vi "Periodic Tasks.vi"(8 "error in":errorcluster) -> ()   [LabVIEW 2015]
doc: "This VI runs in parallel to other tasks. It can contain as many user-defined periodic loops as you need. These can carry out PID or other sorts of timed response."
uses:
  PID Constants.ctl
  DriveTypes.ctl
  <vilib>/Rock Robotics/WPI/DriverStation/WPI_DriverStationAllianceInfo.ctl
  <vilib>/Rock Robotics/WPI/DriverStation/WPI_DriverStationPositionInfo.ctl
  IMUType.ctl
  <userlib>/836-Library/Drive/Drive Code/Drive Code Support/Drive Code PID Bundle.ctl
  <userlib>/836-Library/Pneumatics/Support Code/Solenoid Configure.ctl
  <userlib>/836-Library/Pneumatics/Support Code/Pneumatics Configuration.ctl
  <userlib>/836-Library/Pneumatics/Support Code/Feedback Method.ctl
  <vilib>/Platform/TimedLoop/XDataNode/timing_clust.ctl
  <vilib>/Platform/TimedLoop/XDataNode/nitl_modes.ctl
  <vilib>/Platform/TimedLoop/XDataNode/wakeup.ctl
  <userlib>/836-Library/System/TDMSv2/TDMS Channel Info.ctl
  <userlib>/836-Library/System/TDMSv2/TDMS RT FIFO Packet.ctl
  <vilib>/Rock Robotics/WPI/Utilities/WPI_GetSetVariantRefNum.vi
  <vilib>/Rock Robotics/Network Tables/NT Write Number.vi
  <vilib>/Rock Robotics/Network Tables/NT Write Boolean.vi
  <vilib>/platform/TimedLoop/XDataNode/XDataNode.xnode
  <vilib>/addons/control/pid/NI_PID_pid.lvlib
  <vilib>/Platform/TimedLoop/XDataNode/XDNodeRunTimeDep.lvlib
  <vilib>/addons/control/pid/pid.llb/PID Output Rate Limiter (DBL).vi
panel:
  out "IMU Type":T1
  out "Analog Pitch Gyro 2":dbl(graph)=-229.6875
  in  "Alt imu":bool
  in  "PImu fail":bool
  in  "Reload QCP":bool
  out "Position":T2
  out "Alliance":T3
  in  "Tab Control":enum32{"Drive Test", "IMU", "Drive", "IMU ALT"}(tab)=enum."Drive"
  out "Distance":T4(graph)
  out "Angle":cluster{"Angle Setpoint":dbl, "Yaw":dbl}(graph)={"Angle Setpoint"=87.11416811253483, "Yaw"=3.4375}
  in  "Negates":T5={"negate turn"=TRUE, "negate throttle"=FALSE}
  in  "Throttle Scale":dbl(knob)=0.6332538458134985 scale=0.0..1.0
  in  "Distance Delta":dbl=10.0
  in  "Angle Delta":dbl(knob)=83.67666811253483 scale=-100.0..100.0
  in  "output rate (EGU/min)":dbl(knob)=125.7747299198201 scale=0.0..200.0
  in  "Angle Wrap":bool
  in  "Eval Period (sec)":dbl(knob)=0.503724380465646 scale=0.0..1.0
  in  "tol":dbl=0.5 format="%#_13g"
  out "Shoot":bool
  in  "Period":i64=20
  out "Late?":bool
  out "Delta Angle Remaining":dbl=83.67666811253483
  in  "output range":cluster{"output high":dbl, "output low":dbl}={"output high"=1.0, "output low"=-1.0}
  out "Delta Angle Remaining 3":dbl
  out "Drive Mode 2":T6
  in  "PID Constants":T7={"Drive Distance PID"={"proportional gain (Kc)"=0.2, "integral time (Ti, min)"=0.0, "derivative time (Td, min)"=0.001}, "Drive Straight PID"={"proportional gain (Kc)"=0.035, "integral time (Ti, min)"=0.0, "derivative time (Td, min)"=0.0008}, "TurnPID"={"proportional gain (Kc)"=0.07, "integral time (Ti, min)"=0.005, "derivative time (Td, min)"=0.0008}, "Hold Position PID"={"proportional gain (Kc)"=0.2, "integral time (Ti, min)"=0.02, "derivative time (Td, min)"=0.001}} {"Hold Position PID"."derivative time (Td, min)" format="%.10f"; "Hold Position PID"."integral time (Ti, min)" format="%.8f"; "Hold Position PID"."proportional gain (Kc)" format="%.3f"; "TurnPID"."derivative time (Td, min)" format="%.6f"; "TurnPID"."integral time (Ti, min)" format="%.10f"; "TurnPID"."proportional gain (Kc)" format="%.6f"; "Drive Straight PID"."derivative time (Td, min)" format="%.6f"; "Drive Straight PID"."integral time (Ti, min)" format="%.10f"; "Drive Straight PID"."proportional gain (Kc)" format="%.6f"; "Drive Distance PID"."derivative time (Td, min)" format="%.10f"; "Drive Distance PID"."integral time (Ti, min)" format="%.8f"; "Drive Distance PID"."proportional gain (Kc)" format="%.3f"}
  out "M":T8={"Boolean"=FALSE, "Boolean 2"=FALSE, "Boolean 3"=FALSE, "Boolean 4"=TRUE}
  out "A":T8={"Boolean"=FALSE, "Boolean 2"=FALSE, "Boolean 3"=TRUE, "Boolean 4"=FALSE}
  out "G":T8={"Boolean"=TRUE, "Boolean 2"=FALSE, "Boolean 3"=FALSE, "Boolean 4"=FALSE}
  out "S":T8={"Boolean"=FALSE, "Boolean 2"=FALSE, "Boolean 3"=FALSE, "Boolean 4"=TRUE}
  out "Analog Yaw Gyro":dbl(graph)=-229.6875
  in  "Read Enable":T9={"Cal Status"=TRUE, "Orientation"=TRUE, "Gyro"=FALSE, "Accelerometer"=FALSE, "Quanterion"=FALSE, "Accel Mode"=enum."Linear", "Magnetometer"=FALSE}
  out "Yaw":dbl(graph)=37.4375
  out "Pitch":dbl(graph)=1.75
  out "Roll":dbl(graph)=0.5
  out "X Acc":dbl
  out "Y Acc":dbl
  out "Z Acc":dbl
  out "Anomaly":bool
  in  "Earth Field (uT)":cluster{"Earth":dbl, "Tolerance":dbl}={"Earth"=51.0, "Tolerance"=5.0}
  out "Mag Vector":dbl
  out "IMUStatus":bool
  out "Late? 2":bool
  in  "Sensor Period":i64=20
  out "pitch":dbl=1.75
  in  "Offset 2":dbl(knob)=0.6008653928286186 scale=0.0..1.0
  in  "Dead Zone 2":dbl(knob)=0.09984207295572244 scale=0.0..1.0
  in  "Offset":dbl(knob)=0.267936230826254 scale=0.0..1.0
  in  "Dead Zone":dbl(knob)=0.10126960022109426 scale=0.0..1.0
  out "Left Encoder Distance":dbl=4402.950615
  out "Right Encoder Distance":dbl
  in  "Reset Encoders":bool
  out "pitch 2":dbl=1.75
  out "Mag Vector 2":dbl
  out "Anomaly 2":bool
  in  "Earth Field (uT) 2":cluster{"Earth":dbl, "Tolerance":dbl}={"Earth"=51.0, "Tolerance"=5.0}
  out "Z Acc 2":dbl
  out "Y Acc 2":dbl
  out "X Acc 2":dbl
  out "M 2":T8={"Boolean"=FALSE, "Boolean 2"=FALSE, "Boolean 3"=FALSE, "Boolean 4"=TRUE}
  out "A 2":T8={"Boolean"=FALSE, "Boolean 2"=FALSE, "Boolean 3"=TRUE, "Boolean 4"=FALSE}
  out "G 2":T8={"Boolean"=TRUE, "Boolean 2"=FALSE, "Boolean 3"=FALSE, "Boolean 4"=FALSE}
  out "S 2":T8={"Boolean"=FALSE, "Boolean 2"=FALSE, "Boolean 3"=FALSE, "Boolean 4"=TRUE}
  in  "Read Enable 2":T9={"Cal Status"=TRUE, "Orientation"=TRUE, "Gyro"=FALSE, "Accelerometer"=FALSE, "Quanterion"=FALSE, "Accel Mode"=enum."Linear", "Magnetometer"=FALSE}
  # "Bazemore\nStraight Gains\nP=0.035\nI=0.00\nD=0.0008"
  # "Cass\nHold Position\nGains\nP=0.2\nI=0.02\nD=0.001"
  # "Bazemore\nTurn Gains\nP=0.07\nI=0.005\nD=0.0008"
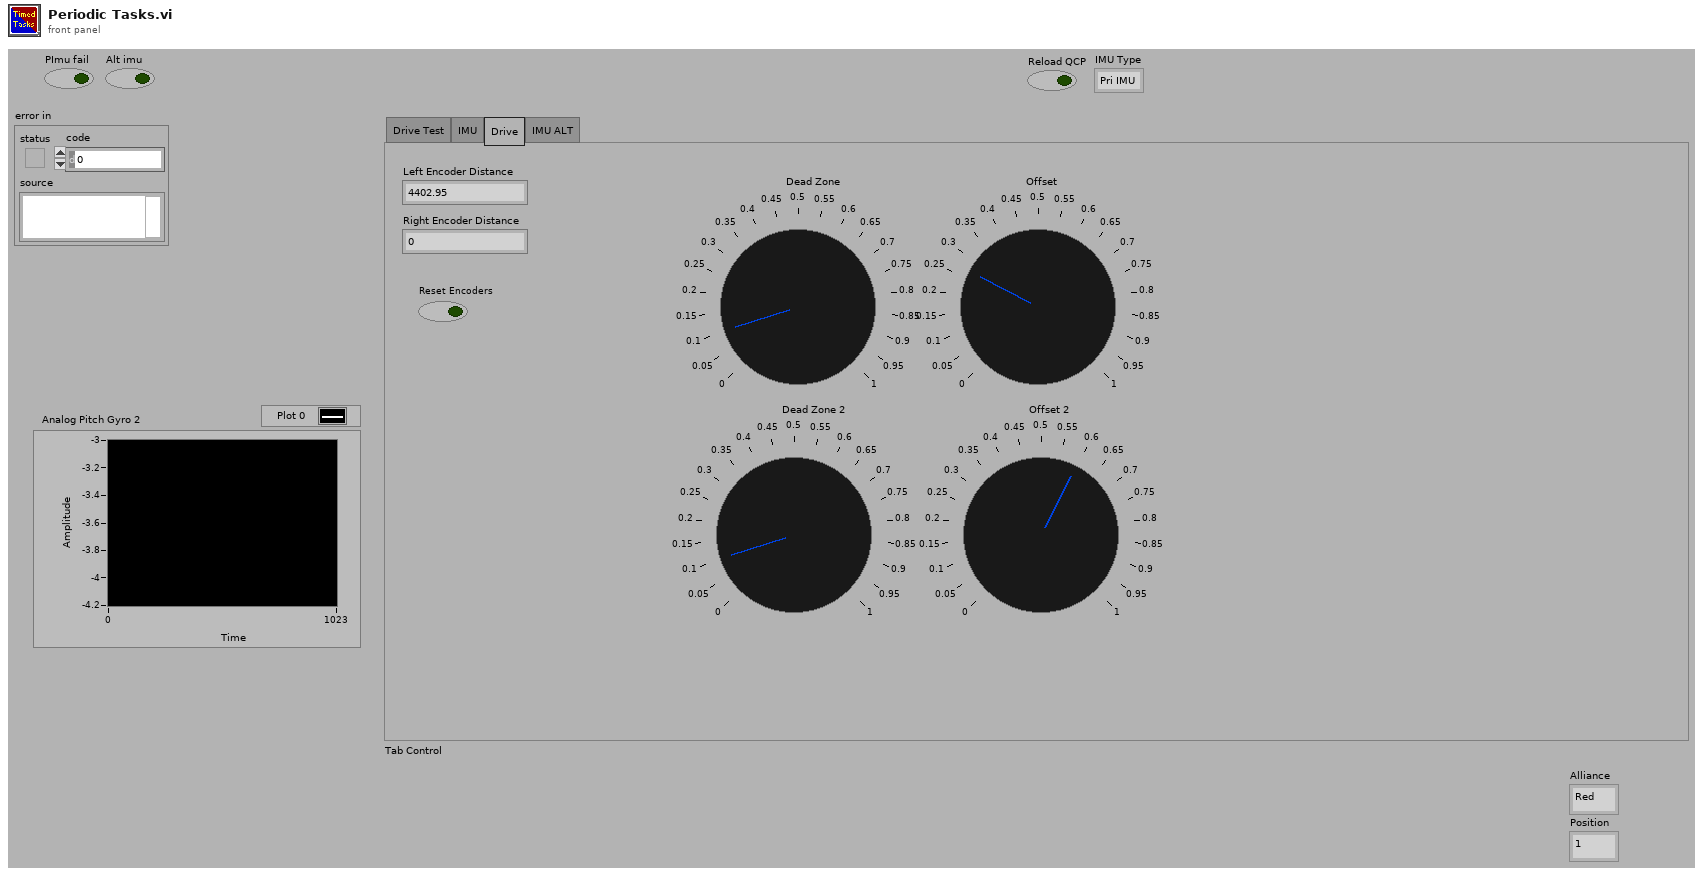
[diagram p1: front panel]
types:
  T1 = typedef "IMUType.ctl" = enum16{"Pri IMU", "Alt IMU", "Analog GYRO"}
  T2 = typedef "WPI_DriverStationPositionInfo.ctl" = enum16{"1", "2", "3"}
  T3 = typedef "WPI_DriverStationAllianceInfo.ctl" = enum16{"Red", "Blue", "Invalid"}
  T4 = cluster{"Distance Setpoint":dbl, "Desired Distance":dbl}
  T5 = cluster{"negate turn":bool, "negate throttle":bool}
  T6 = typedef "DriveTypes.ctl" = enum16{"Auto Turn", "Auto Straight", "Auto Vision Align"}
  T7 = typedef "PID Constants.ctl" = cluster{"Drive Distance PID":cluster{"proportional gain (Kc)":dbl, "integral time (Ti, min)":dbl, "derivative time (Td, min)":dbl}, "Drive Straight PID":cluster{"proportional gain (Kc)":dbl, "integral time (Ti, min)":dbl, "derivative time (Td, min)":dbl}, "TurnPID":cluster{"proportional gain (Kc)":dbl, "integral time (Ti, min)":dbl, "derivative time (Td, min)":dbl}, "Hold Position PID":cluster{"proportional gain (Kc)":dbl, "integral time (Ti, min)":dbl, "derivative time (Td, min)":dbl}}
  T8 = cluster{"Boolean":bool, "Boolean 2":bool, "Boolean 3":bool, "Boolean 4":bool}
  T9 = cluster{"Cal Status":bool, "Orientation":bool, "Gyro":bool, "Accelerometer":bool, "Quanterion":bool, "Accel Mode":enum8{"Raw Data", "Linear", "Gravity"}, "Magnetometer":bool}
  T10 = cluster{"Group":string, "Channel Names":string[]}[]
  T11 = typedef "TDMS Channel Info.ctl" = cluster{"TDMS Data":T12, "TDMS RT FIFO":refnum<k33>}
  T12 = typedef "TDMS RT FIFO Packet.ctl" = cluster{"Group/CMD":i32, "Channel":i32, "Data":dbl}
  T13 = cluster{"IMU Yaw":T11, "IMU Pitch":T11, "IMU Roll":T11, "Accel X":T11, "Accel Y":T11, "Accel Z":T11, "IMU Cal M":T11, "IMU Cal A":T11, "IMU Cal G":T11, "IMU Cal S":T11, "IMU Type":T11}
  T14 = typedef "Solenoid Configure.ctl" = cluster{"Normal Timing":T15, "Feedback Forward":T16, "Feedback Reverse":T16, "Analog Thresholds":T15, "Timeout":T15}
  T15 = typedef "Pneumatics Configuration.ctl" = cluster{"Forward":dbl, "Reverse":dbl}
  T16 = typedef "Feedback Method.ctl" = enum16{"Timed", "Analog", "Digital", "Analog (Inverted)", "Digital (Inverted)"}
  T17 = typedef "Drive Code PID Bundle.ctl" = cluster{"Yaw, Driving Straight":cluster{"proportional gain (Kc)":dbl, "integral time (Ti, min)":dbl, "derivative time (Td, min)":dbl}, "Yaw, Holding Still":cluster{"proportional gain (Kc)":dbl, "integral time (Ti, min)":dbl, "derivative time (Td, min)":dbl}, "Distance, Driving Straight":cluster{"proportional gain (Kc)":dbl, "integral time (Ti, min)":dbl, "derivative time (Td, min)":dbl}, "Distance, Holding Still":cluster{"proportional gain (Kc)":dbl, "integral time (Ti, min)":dbl, "derivative time (Td, min)":dbl}}
  T18 = cluster{"Yaw Wind":dbl, "Roll Wind":dbl, "Pitch Wind":dbl}
  T19 = typedef "Drive Code Bundle.ctl" = cluster{"Sensor Data":T20, "Drive Command rt fifo":refnum<k33>, "Logging Data":refnum<k33>}
  T20 = typedef "Sensor Cluster.ctl" = cluster{"Gyro Data":cluster{"Gyro RT FIFO":refnum<k33>, "Gyro Current":dbl, "Gyro Hold":dbl}, "Encoder Data":cluster{"Encoder RT FIFO":refnum<k33>, "Encoder Current":dbl, "Encoder Hold":dbl}, "Camera Data":cluster{"Camera RT FIFO":refnum<k33>, "Camera Current":T21}}
  T21 = typedef "Camera Cluster.ctl" = cluster{" Angle":dbl, "Valid":bool}
  T22 = cluster{"proportional gain (Kc)":dbl, "integral time (Ti, min)":dbl, "derivative time (Td, min)":dbl}
  T23 = typedef "XDNodeRunTimeDep.lvlib/timing_clust.ctl" = cluster{"Expected End [f-1]":u64, "Actual End [f-1]":u64, "Finished Late? [f-1]":bool, "Expected End [i-1]":u64, "Actual End [i-1]":u64, "Finished Late? [i-1]":bool, "Expected Start [i]":u64, "Actual Start [i]":u64, "Expected Start [f]":u64, "Actual Start [f]":u64, "Source Name":string, "Structure Name":string, "Period":i64, "Deadline":i64, "Offset":i64, "Start":i64, "Priority":i32, "Timeout":i32, "Mode":T24, "Wakeup Reason":T25, "Error":errorcluster, "Source Type":string, "Secondary Source Type":string, "Global End Time":u64, "Global Start Time":u64, "Frame Duration":u64, "Iteration Duration":u64, "Assigned CPU":i32, "I/O Scan Engine Mode":u32}
  T24 = typedef "XDNodeRunTimeDep.lvlib/nitl_modes.ctl" = enum32{"No Change", "Process missed periods, maintain original phase", "Discard missed periods, maintain original phase", "Process missed periods, ignore original phase", "Discard missed periods, ignore original phase"}
  T25 = typedef "XDNodeRunTimeDep.lvlib/wakeup.ctl" = enum32{"Normal", "Aborted", "Asynchronous wakeup", "Timing source error", "Timed loop error", "Timeout"}
  T26 = cluster{"Delta":dbl, "Throttle Scale":dbl, "Current Angle":dbl, "Current Distance":dbl}
  T27 = typedef "WPI_RobotDriveDevRef.ctl" = cluster{"DevStatus":errorcluster, "Motors[]":T28[], "Square Inputs":bool, "Max Output":dbl}
  T28 = typedef "WPI_MotorControlDeviceRef.ctl" = cluster{"DeviceStatus":errorcluster, "Type":T29, "PWM":cluster{"PWM Channel":T30, "DeadBand":T31}, "CAN":cluster{"Device Number":u8, "Control Mode":T32, "Semaphore":T33, "Max Vout":dbl, "TalonSRX Control Mode":T34}, "Invert":bool}
  T29 = typedef "WPI_MotorControlType.ctl" = enum16{"PWM", "CAN", "CANTalonSRX"}
  T30 = typedef "FPGA_DIOPWMChannel.ctl" = enum8{"PWM 0", "PWM 1", "PWM 2", "PWM 3", "PWM 4", "PWM 5", "PWM 6", "PWM 7", "PWM 8", "PWM 9", "PWM MXP 0", "PWM MXP 1", "PWM MXP 2", "PWM MXP 3", "PWM MXP 4", "PWM MXP 5", "PWM MXP 6", "PWM MXP 7", "PWM MXP 8", "PWM MXP 9", "Invalid"}
  T31 = typedef "WPI_PWMDeadband.ctl" = cluster{"Name":string, "maxPositivePwm":i32, "minPositivePwm":i32, "centerPwm":i32, "maxNegativePwm":i32, "minNegativePwm":i32, "angularRange":u16}
  T32 = typedef "WPI_CANJaguar_ControlMode.ctl" = enum8{"Percent VBus", "Current", "Speed", "Position", "Voltage"}
  T33 = typedef "Semaphore RefNum" = refnum<k1>
  T34 = typedef "WPI_CANTalonSRX_APIControlMode.ctl" = enum8{"Percent VBus", "Speed", "Position", "Slave", "Unchanged / Invalid", "Voltage Compensation", "Current", "Motion Profile"}
  T35 = typedef "WPI_JoystickDevRef.ctl" = cluster{"Device":T36}
  T36 = typedef "WPI_JoystickDeviceEnum.ctl" = enum16{"USB 0", "USB 1", "USB 2", "USB 3", "USB 4", "USB 5"}
  T37 = cluster{"Buttons[0]":bool, "Buttons[1]":bool, "Buttons[2]":bool, "Buttons[3]":bool, "Buttons[4]":bool, "Buttons[5]":bool, "Buttons[6]":bool, "Buttons[7]":bool, "Buttons[8]":bool}
  T38 = cluster{"Axes[0]":dbl, "Axes[1]":dbl, "Axes[2]":dbl, "Axes[3]":dbl, "Axes[4]":dbl, "Axes[5]":dbl, "Axes[6]":dbl, "Axes[7]":dbl, "Axes[8]":dbl}
  T39 = cluster{"Drive Distance PID":cluster{"proportional gain (Kc)":dbl, "integral time (Ti, min)":dbl, "derivative time (Td, min)":dbl}, "Drive Straight PID":cluster{"proportional gain (Kc)":dbl, "integral time (Ti, min)":dbl, "derivative time (Td, min)":dbl}}
  T40 = cluster{"Angle Setpoint":dbl, "Distance Setpoint":dbl}
  T41 = cluster{"Distance Setpoint":dbl, "Current Distance":dbl}
  T42 = typedef "Logging Data.ctl" = cluster{"Command":T43, "Desired Angle":dbl, "Desired Encoder":dbl}
  T43 = typedef "Drive Code Command.ctl" = enum16{"Do Nothing", "Manual", "Drive Continuous", "Turn", "Drive Distance", "Hold Position", "Hold Yaw", "Follow Camera", "Turn to Camera"}
  T44 = typedef "WPI_SolenoidDevRef.ctl" = cluster{"DevStatus":errorcluster, "Pneumatics Control Module":u8, "Forward Solenoid Channel":T45, "Reverse Solenoid Channel":T45}
  T45 = typedef "WPI_SolenoidChannel.ctl" = enum8{"Solenoid 0", "Solenoid 1", "Solenoid 2", "Solenoid 3", "Solenoid 4", "Solenoid 5", "Solenoid 6", "Solenoid 7", "Invalid"}
  T46 = typedef "Pneumatic Sensor Loop.ctl" = cluster{"Status Queue":refnum<queue>, "Status Loop":refnum<k33>, "Relay Value":T47}
  T47 = typedef "WPI_SolenoidValue.ctl" = enum16{"Off", "On", "Forward", "Reverse"}
  T48 = typedef "Solenoid Control Loop.ctl" = cluster{"Control Notifier":refnum<notifier>, "Initial Position":T49, "SolenoidDevRef":T44, "Status Loop":refnum<k33>}
  T49 = typedef "Pneumatics Position.ctl" = enum16{"Forward", "Reverse"}
  T50 = typedef "WPI_EncoderDevRef.ctl" = cluster{"DevStatus":errorcluster, "EncoderIndex":T51, "CounterIndex":T52, "DistancePerCount":dbl, "Decoding Type":T53}
  T51 = typedef "FPGA_EncoderIdx.ctl" = enum8{"Enc 0", "Enc 1", "Enc 2", "Enc 3", "Enc 4", "Enc 5", "Enc 6", "Enc 7", "Invalid"}
  T52 = typedef "FPGA_CounterCtrSystemIndex.ctl" = enum8{"Ctr 0", "Ctr 1", "Ctr 2", "Ctr 3", "Ctr 4", "Ctr 5", "Ctr 6", "Ctr 7", "Invalid"}
  T53 = typedef "WPI_EncoderType.ctl" = enum16{"1x", "2x", "4x"}
  T54 = typedef "WPI_GyroDevRef.ctl" = cluster{"DevStatus":errorcluster, "Analog Channel":T55, "Offset":dbl, "Gain (VoltsPerDegree/Second)":dbl, "Gyro Type":enum16{"Analog", "XRS450"}, "Handle":i32, "SPI Bus":T56, "Device Found":bool, "Sample Rate":dbl, "Calibrate On Open":bool}
  T55 = typedef "FPGA_AIChannel.ctl" = enum8{"AI 0", "AI 1", "AI 2", "AI 3", "AI MXP 0", "AI MXP 1", "AI MXP 2", "AI MXP 3", "Invalid"}
  T56 = typedef "spi_bus.ctl" = enum16{"SPI On-Board, CS0", "SPI On-Board, CS1", "SPI On-Board, CS2", "SPI On-Board, CS3", "SPI MXP", "Invalid"}
  T57 = typedef "WPI_I2CDevRef.ctl" = cluster{"DevStatus":errorcluster, "Device Address":u8, "Handle":i32, "I2C Bus":T58}
  T58 = typedef "i2c_bus.ctl" = enum16{"I2C On-Board", "I2C MXP", "Invalid"}
  T59 = cluster{"Mag":cluster{"[0]":bool, "[1]":bool, "[2]":bool, "[3]":bool}, "Acc":cluster{"[0]":bool, "[1]":bool, "[2]":bool, "[3]":bool}, "Gyro":cluster{"[0]":bool, "[1]":bool, "[2]":bool, "[3]":bool}, "Sys":cluster{"[0]":bool, "[1]":bool, "[2]":bool, "[3]":bool}, "Status":bool}
  T60 = cluster{"Yaw":dbl, "Roll":dbl, "Pitch":dbl, "Yaw Wind":dbl, "Roll Wind":dbl, "Pitch Wind":dbl}
  T61 = cluster{"X Mag":dbl, "Y Mag":dbl, "Z Mag":dbl, "Anomaly":bool}
  T62 = cluster{"[0]":bool, "[1]":bool, "[2]":bool, "[3]":bool}
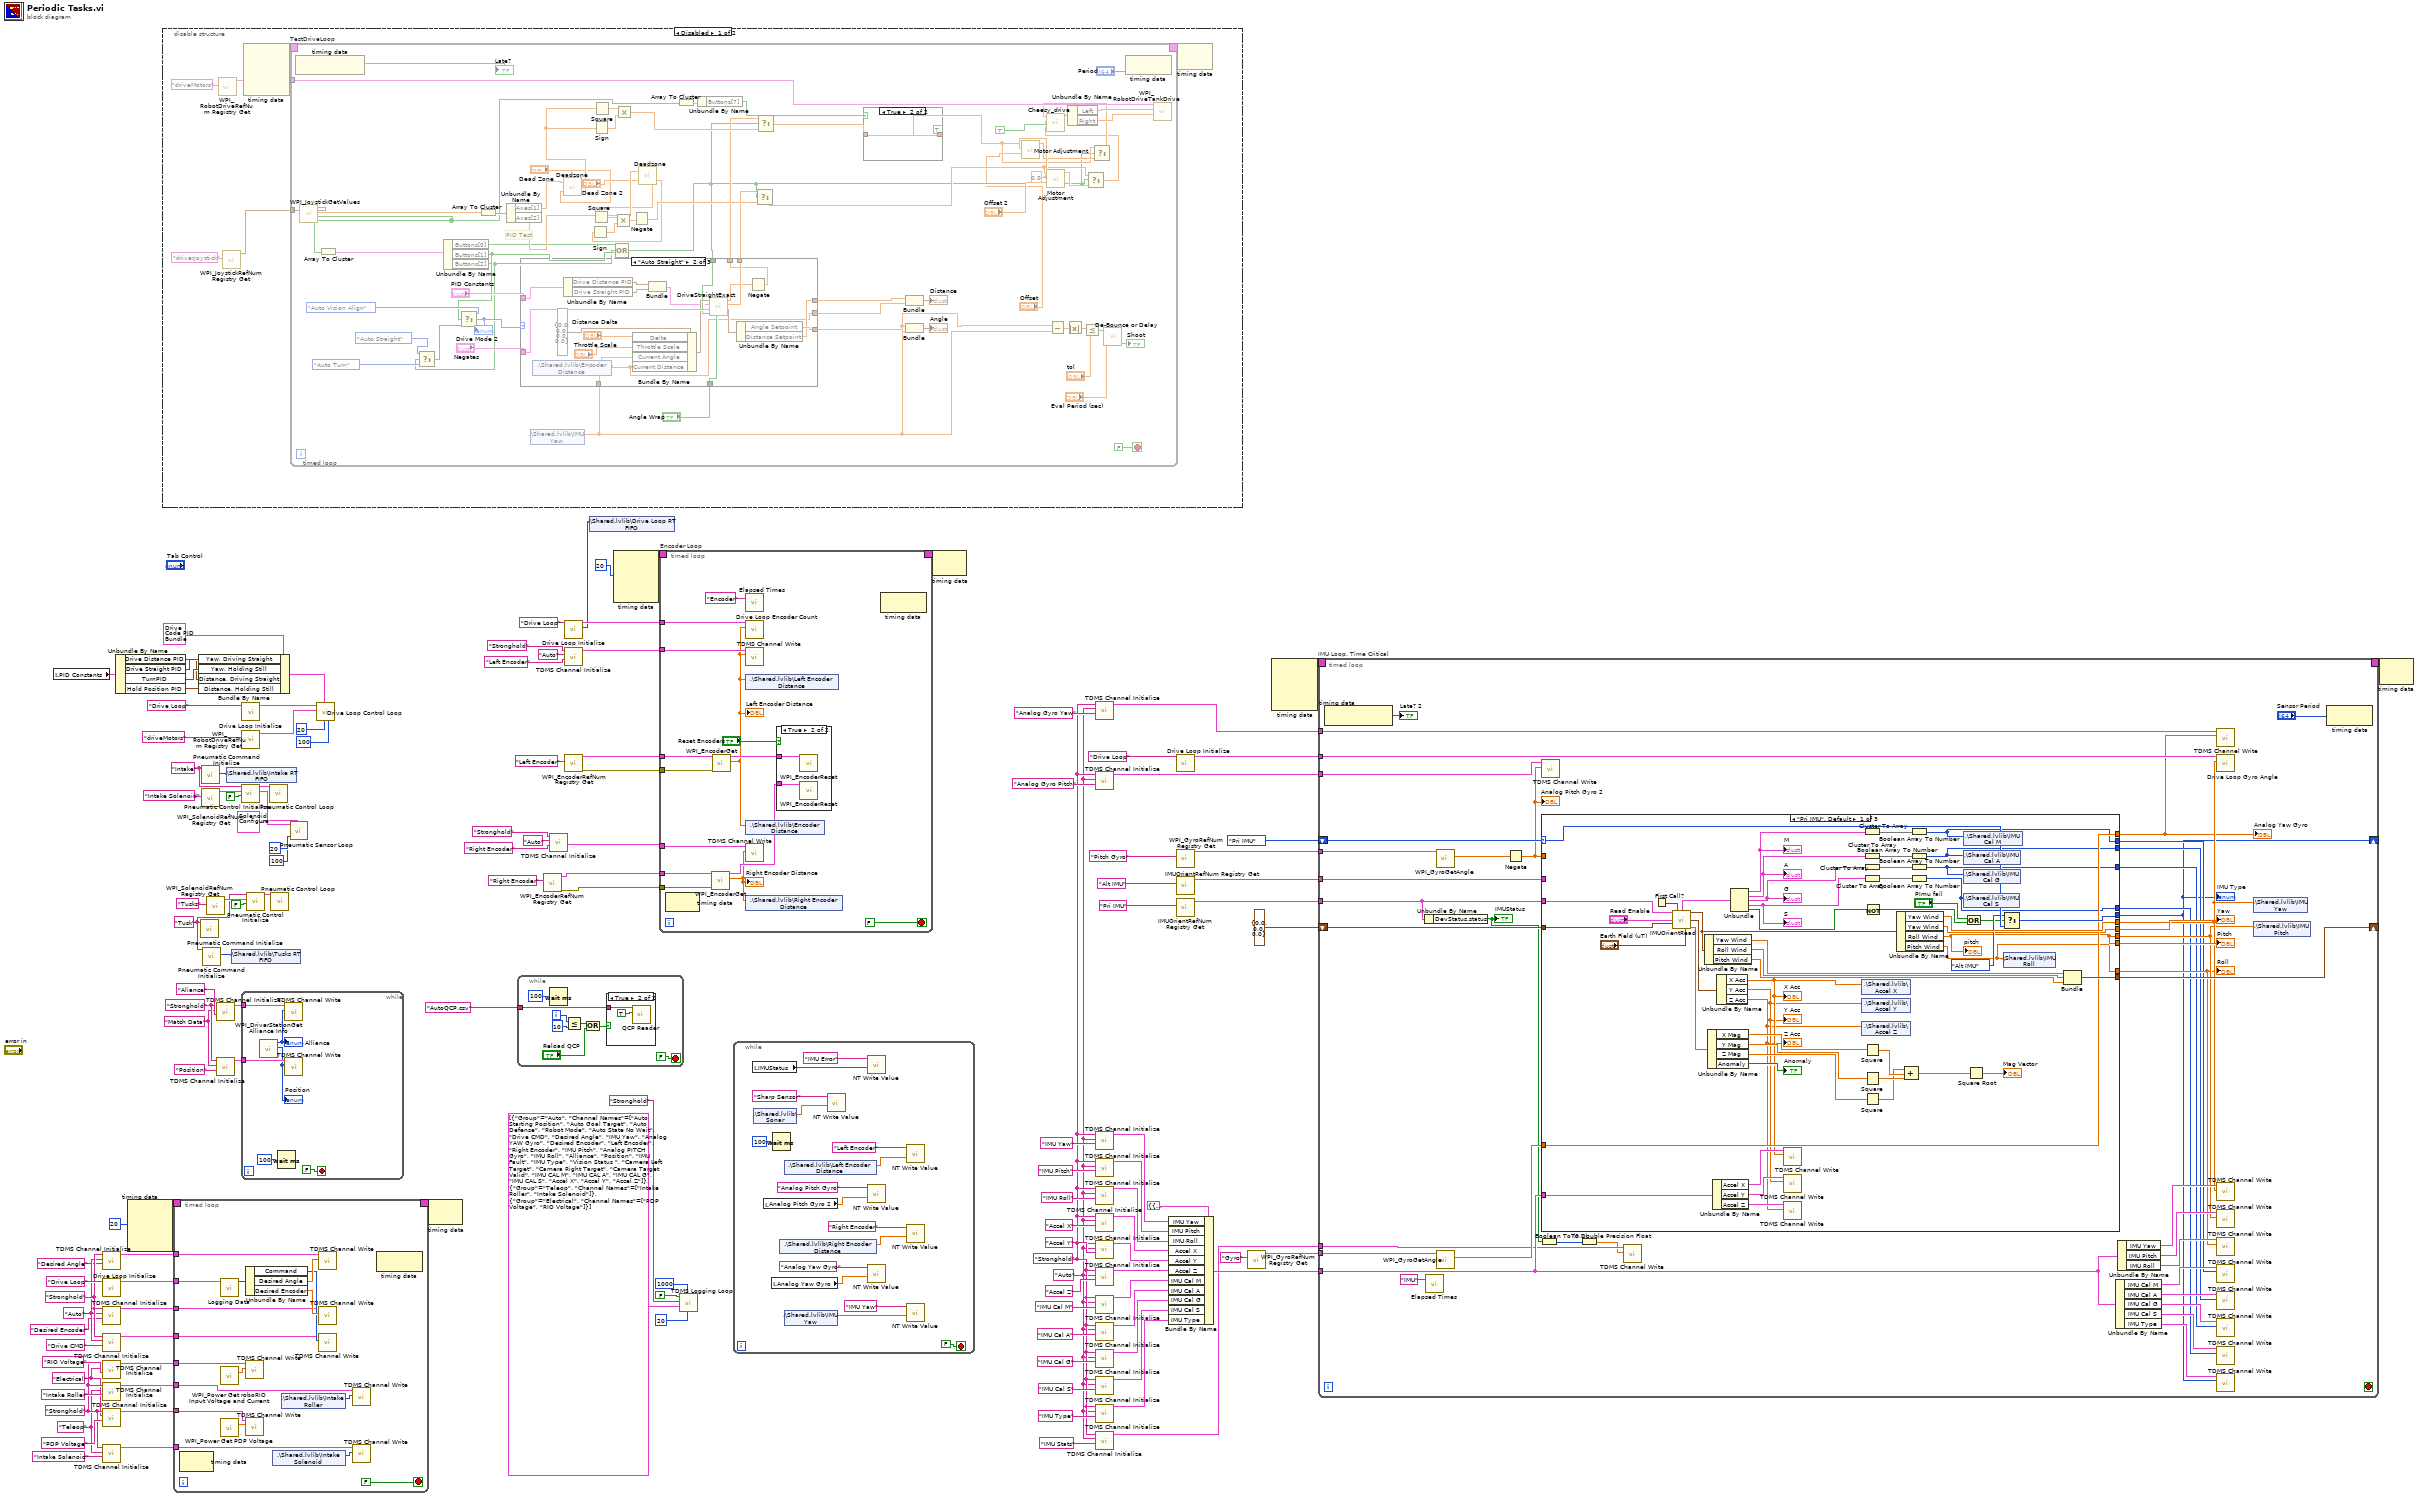
[diagram p0: block diagram]
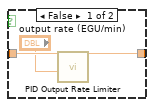
[diagram p2: hidden frame]
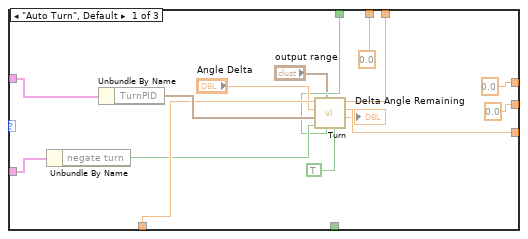
[diagram p3: hidden frame]
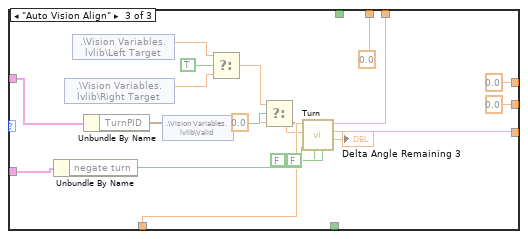
[diagram p4: hidden frame]
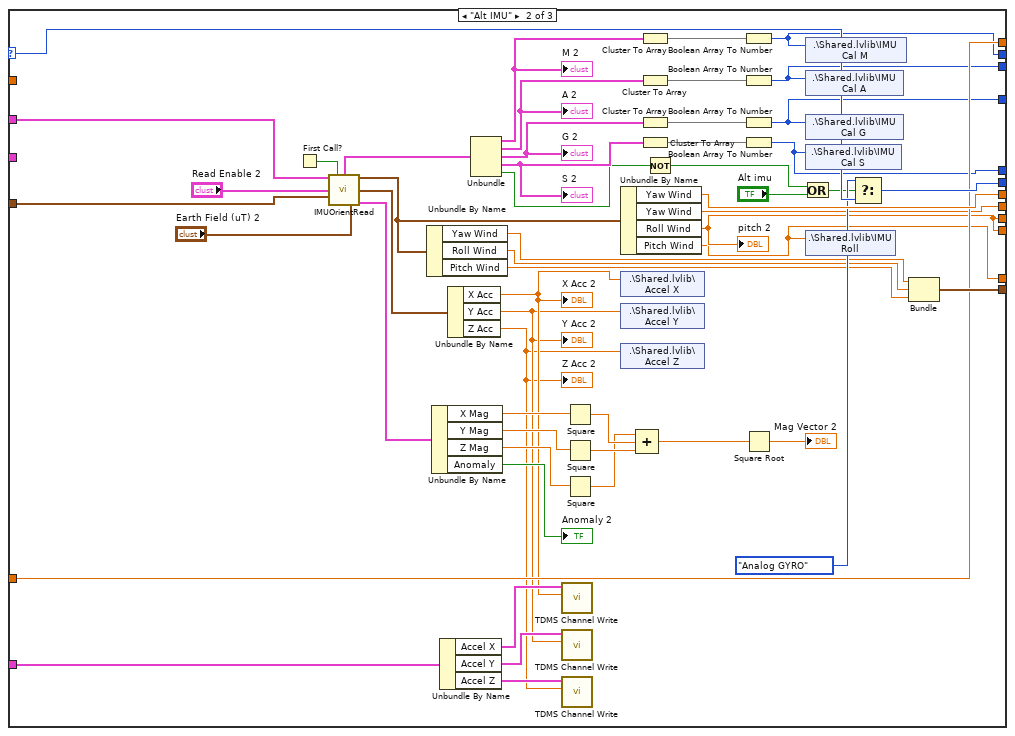
[diagram p8: hidden frame]
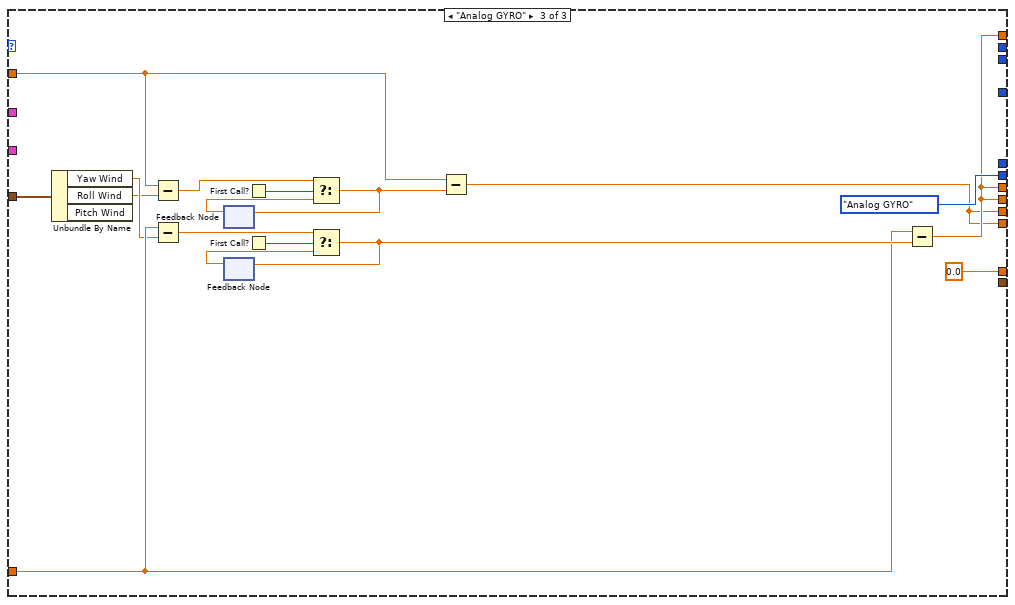
[diagram p9: hidden frame]
diagram:
  w6 = "Auto" ("Group")
  w7 = "Stronghold" ("TDMS")
  w15 = "Stronghold" ("TDMS")
  w14 = "Match Data" ("TDMS")
  w18 = "Electrical" ("Group")
  w17 = "Teleop" ("Group")
  w19 = "Stronghold" ("TDMS")
  w32 = "Auto" ("Group")
  w33 = "Stronghold" ("TDMS Name")
  w77 = "Intake" ("name (unnamed)")
  w85 = "Tusk" ("name (unnamed)")
  n1 = local read "PID Constants"() -> (w98:T7)
  n2 = call <userlib>:"TDMS Channel Initialize.vi"("Channel"="Desired Angle", "Group"=w6, "TDMS"=w7) -> ("TDMS Channel Info"=w2:T11)  [unwired: 8 in]
  n3 = call <userlib>:"Drive Loop Initialize.vi"("name (unnamed)"="Drive Loop") -> ("Drive Loop Cluster"=w9:T19)  [unwired: 9 in, 1 out]
  n4 = call <userlib>:"TDMS Channel Initialize.vi"("Channel"="Desired Encoder", "Group"=w6, "TDMS"=w7) -> ("TDMS Channel Info"=w1:T11)  [unwired: 8 in]
  n5 = call <userlib>:"TDMS Channel Initialize.vi"("Channel"="Drive CMD", "Group"=w6, "TDMS"=w7) -> ("TDMS Channel Info"=w3:T11)  [unwired: 8 in]
  n6 = call <userlib>:"TDMS Channel Initialize.vi"("Channel"="RIO Voltage", "Group"=w18, "TDMS"=w19) -> ("TDMS Channel Info"=w20:T11)  [unwired: 8 in]
  n7 = call <userlib>:"TDMS Channel Initialize.vi"("Channel"="Intake Roller", "Group"=w17, "TDMS"=w19) -> ("TDMS Channel Info"=w24:T11)  [unwired: 8 in]
  n8 = call <userlib>:"TDMS Channel Initialize.vi"("Channel"="PDP Voltage", "Group"=w18, "TDMS"=w19) -> ("TDMS Channel Info"=w21:T11)  [unwired: 8 in]
  n9 = call <userlib>:"TDMS Channel Initialize.vi"("Channel"="Intake Solenoid", "Group"=w17, "TDMS"=w19) -> ("TDMS Channel Info"=w25:T11)  [unwired: 8 in]
  n10 = Unbundle By Name(w98) -> ("Drive Distance PID"=w95:T22, "Drive Straight PID"=w96:T22, "TurnPID"=w97:T22, "Hold Position PID"=w94:T22)
  n11 = node-c288(i64 20 ("Period")) -> (w28:T23)  [unwired: 3 in]
  n12 = disable-structure shown="Disabled" {
    frame Disabled {
      n13 = call <vilib>:"WPI_RobotDriveRefNum Registry Get.vi"("refnum name"="driveMotors") -> ("RobotDriveDevRef"=w134:T27)  [unwired: 9 in, 1 out]
      n14 = call <vilib>:"WPI_JoystickRefNum Registry Get.vi"("refnum name"="driverJoystick") -> ("JoystickDevRef"=w132:T35)  [unwired: 9 in, 1 out]
      n15 = node-c288() -> (w137:T23)  [unwired: 4 in]
      n16 = timed-loop "TestDriveLoop" {
        tunnel: w134 -> [w197]
        tunnel: w132 -> [w201]
        timing: w137 -> [_]
        timing-out: [_] -> w136
        stop <- FALSE stop-if-true
        w155 = 0.0 ("Dead Zone")
        (unwired) TRUE ("Quick Turn")
        # "PID Test"
        n17 = node-c288() -> (→"Late?":bool)  [unwired: 1 in]
        n18 = call <vilib>:"WPI_JoystickGetValues.vi"("JoystickDevRef"=w201) -> ("Buttons"=w175:bool[], "Axes"=w200:dbl[])  [unwired: 6 in, 3 out]
        n19 = Array To Cluster(array=w175) -> (cluster=w191:T37)
        n20 = Unbundle By Name(w191) -> ("Buttons[0]"=w141:bool, "Buttons[1]"=w158:bool, "Buttons[2]"=w156:bool)
        n21 = Select(t=DriveTypes."Auto Straight", s=w156, f=DriveTypes."Auto Turn") -> (s? t:f=w159:T6)
        n22 = Select(t=DriveTypes."Auto Vision Align", s=w158, f=w159) -> (s? t:f=w162:T6)
        "Drive Mode 2" <- w162
        n23 = Array To Cluster(array=w200) -> (cluster=w199:T38)
        n24 = Unbundle By Name(w199) -> ("Axes[1]"=w154:dbl, "Axes[2]"=w152:dbl)
        n25 = shared-variable ".\\Shared.lvlib\\IMU Yaw"() -> (w163:dbl)  [unwired: 1 in, 1 out]
        n26 = call <userlib>:"Deadzone.vi"("Deadzone"="Dead Zone", "Input Signal"=w154) -> ("Output Signal"=w153:dbl)  [unwired: 1 out]
        n27 = Sign(1:w153) -> (0:w193:dbl)
        n28 = Square(x=w153) -> (x^2=w192:dbl)
        n29 = Multiply(x=w192, y=w193) -> (x*y=w180:dbl)
        n30 = Compound Arithmetic op=OR(w141, w156, w158) -> (w140:bool)
        n31 = case shown="\"Auto Straight\"" w162 {
          tunnel: [w217 w243 w254] -> w170
          tunnel: w163 -> [w223 w242 w262]
          tunnel: [0.0 ("Distance Setpoint") w241 0.0 ("Distance Setpoint")] -> w188
          tunnel: [0.0 ("Current Distance") w232 0.0 ("Current Distance")] -> w187
          tunnel: "PID Constants" -> [w225 w229 w258]
          tunnel: "Negates" -> [w221 w238 w264]
          tunnel: [w219 w237 w253] -> w179
          tunnel: [0.0 ("Cheesy Throttle") w230 0.0 ("Cheesy Throttle")] -> w178
          tunnel: "Angle Wrap" -> [_ w234 _]
          tunnel: w140 -> [w214 w233 _]
          frame "Auto Turn", Default {
            n32 = Unbundle By Name(w221) -> ("negate turn"=w220:bool)
            n33 = Unbundle By Name(w225) -> ("TurnPID"=w224:T22)
            n34 = call "Turn.vi"("Delta?"=TRUE, "Start Turn"=w214, "output range"="output range", "Negate"=w220, "PID gains"=w224, "Desired Angle"="Angle Delta", "Current Angle"=w223) -> ("Delta Angle Remaining"=→"Delta Angle Remaining":dbl, "Setpoint"=w217:dbl, "Cheesy Steer"=w219:dbl)  [unwired: 1 in, 1 out]
          }
          frame "Auto Straight" {
            n35 = shared-variable ".\\Shared.lvlib\\Encoder Distance"() -> (w232:dbl)  [unwired: 1 in, 1 out]
            n36 = Unbundle By Name(w229) -> ("Drive Distance PID"=w228:T22, "Drive Straight PID"=w227:T22)
            n37 = Bundle By Name(cluster=T26 {"Delta"=0.0, "Throttle Scale"=0.0, "Current Angle"=0.0, "Current Distance"=0.0} ("Drive Values"), "Delta"="Distance Delta", "Throttle Scale"="Throttle Scale", "Current Angle"=w242, "Current Distance"=w232) -> (w235:T26)
            n38 = Bundle("Drive Distance PID"=w228, "Drive Straight PID"=w227) -> (w226:T39)  [unwired: 1 in]
            n39 = call "DriveStraightExact.vi"("Angle Wrap"=w234, "Start Drive Straight (Hold)"=w233, "Negates"=w238, "PID Constants"=w226, "Drive Values"=w235) -> ("Setpoints"=w239:T40, "Cheesy Steer"=w237:dbl, "Cheesy Throttle"=w231:dbl)  [unwired: 4 in]
            n40 = Unbundle By Name(w239) -> ("Angle Setpoint"=w243:dbl, "Distance Setpoint"=w241:dbl)
            n41 = Negate(x=w231) -> (-x=w230:dbl)
          }
          frame "Auto Vision Align" {
            n42 = Unbundle By Name(w264) -> ("negate turn"=w263:bool)
            n43 = shared-variable ".\\Vision Variables.lvlib\\Right Target"() -> (w249:dbl)  [unwired: 1 in, 1 out]
            n44 = shared-variable ".\\Vision Variables.lvlib\\Left Target"() -> (w250:dbl)  [unwired: 1 in, 1 out]
            n45 = Unbundle By Name(w258) -> ("TurnPID"=w257:T22)
            n46 = shared-variable ".\\Vision Variables.lvlib\\Valid"() -> (w260:bool)  [unwired: 1 in, 1 out]
            n47 = Select(t=w250, s=TRUE, f=w249) -> (s? t:f=w248:dbl)
            n48 = Select(t=w248, s=w260, f=0.0) -> (s? t:f=w261:dbl)
            n49 = call "Turn.vi"("Delta?"=FALSE, "Start Turn"=FALSE, "Negate"=w263, "PID gains"=w257, "Desired Angle"=w261, "Current Angle"=w262) -> ("Delta Angle Remaining"=→"Delta Angle Remaining 3":dbl, "Setpoint"=w254:dbl, "Cheesy Steer"=w253:dbl)  [unwired: 2 in, 1 out]
          }
        }
        n50 = call <userlib>:"Deadzone.vi"("Deadzone"="Dead Zone 2", "Input Signal"=w152) -> ("Output Signal"=w151:dbl)  [unwired: 1 out]
        n51 = Sign(1:w151) -> (0:w195:dbl)
        n52 = Square(x=w151) -> (x^2=w196:dbl)
        n53 = Multiply(x=w196, y=w195) -> (x*y=w194:dbl)
        n54 = Negate(x=w194) -> (-x=w181:dbl)
        n55 = Array To Cluster(array=w175) -> (cluster=w176:T37)
        n56 = Unbundle By Name(w176) -> ("Buttons[7]"=w174:bool)
        n57 = Select(t=w179, s=w140, f=w181) -> (s? t:f=w142:dbl)
        n58 = Select(t=w178, s=w140, f=w180) -> (s? t:f=w177:dbl)
        n59 = case shown="True" w174 {
          tunnel: [w209 w210] -> w143
          tunnel: w177 -> [w208 w210]
          frame False {
            n60 = call-poly <vilib>:"PID Output Rate Limiter.vi"("output rate (EGU/min)"="output rate (EGU/min)", "input (controller output)"=w208) -> ("output"=w209:dbl)  [unwired: 6 in, 1 out]
          }
          frame True {
          }
        }
        n61 = Bundle("Distance Setpoint"=w188, "Current Distance"=w187) -> (→"Distance":T41)  [unwired: 1 in]
        n62 = Bundle("Setpoint"=w170, "Double"=w163) -> (→"Angle":cluster{"Setpoint":dbl, "Double":dbl})  [unwired: 1 in]
        n63 = call "Motor Adjustment.vi"("Offset"="Offset", "Dead Zone"=w155, "X in"=w143) -> ("X Out"=w144:dbl)  [unwired: 8 in]
        n64 = call "Motor Adjustment.vi"("Offset"="Offset 2", "Dead Zone"=w155, "X in"=w142) -> ("X Out"=w145:dbl)  [unwired: 8 in]
        n65 = Subtract(x=w170, y=w163) -> (x-y=w169:dbl)
        n66 = Absolute Value(x=w169) -> (abs(x)=w168:dbl)
        n67 = Less Or Equal?(x=w168, y="tol") -> (x <= y?=w166:bool)
        n68 = Select(t=w142, s=w140, f=w145) -> (s? t:f=w146:dbl)
        n69 = Select(t=w143, s=w140, f=w144) -> (s? t:f=w147:dbl)
        n70 = call "Cheesy_drive.vi"("Quick Turn"=TRUE, "Wheel"=w146, "Throttle"=w147) -> ("Drive Data"=w184:cluster{"Left":dbl, "Right":dbl})  [unwired: 8 in]
        n71 = Unbundle By Name(w184) -> ("Left"=w183:dbl, "Right"=w182:dbl)
        n72 = call <userlib>:"De-Bounce or Delay.vi"("Eval Period (sec)"="Eval Period (sec)", "Signal Input"=w166) -> ("Stable"=→"Shoot":bool)  [unwired: 9 in]
        n73 = node-c288("Period") -> ()  [unwired: 1 out]
        n74 = call <vilib>:"WPI_RobotDriveTankDrive.vi"("Right axis value"=w182, "Left axis value"=w183, "RobotDriveDevRef"=w197) -> ()  [unwired: 6 in, 3 out]
      }
      n75 = node-c288(w136) -> ()  [unwired: 1 out]
    }
    frame Enabled {
    }
  }
  n76 = timed-loop {
    timing: w28 -> [_]
    timing-out: [_] -> w27
    tunnel: w25 -> [w282]
    tunnel: w24 -> [w281]
    tunnel: w21 -> [w278]
    tunnel: w20 -> [w277]
    tunnel: w9 -> [w274]
    tunnel: w3 -> [w269]
    tunnel: w2 -> [w268]
    tunnel: w1 -> [w267]
    stop <- FALSE stop-if-true
    n77 = node-c288() -> ()  [unwired: 1 in, 1 out]
    n78 = call <userlib>:"Logging Data.vi"("Drive Loop Cluster"=w274) -> ("Logging Data"=w273:T42)  [unwired: 10 in]
    n79 = call <vilib>:"WPI_Power Get roboRIO Input Voltage and Current.vi"() -> ("roboRIO input voltage (V)"=w276:dbl)  [unwired: 13 in, 2 out]
    n80 = call <vilib>:"WPI_Power Get PDP Voltage.vi"() -> ("voltage (V)"=w275:dbl)  [unwired: 14 in, 1 out]
    n81 = Unbundle By Name(w273) -> ("Command"=w270:T43, "Desired Angle"=w271:dbl, "Desired Encoder"=w272:dbl)
    n82 = call <userlib>:"TDMS Channel Write.vi"("Data"=w276, "TDMS Channel Info in"=w277) -> ()  [unwired: 9 in, 1 out]
    n83 = call <userlib>:"TDMS Channel Write.vi"("Data"=w275, "TDMS Channel Info in"=w278) -> ()  [unwired: 9 in, 1 out]
    n84 = shared-variable ".\\Shared.lvlib\\Intake Solenoid"() -> (w280:u32)  [unwired: 1 in, 1 out]
    n85 = shared-variable ".\\Shared.lvlib\\Intake Roller"() -> (w279:u32)  [unwired: 1 in, 1 out]
    n86 = call <userlib>:"TDMS Channel Write.vi"("Data"=w271, "TDMS Channel Info in"=w268) -> ()  [unwired: 9 in, 1 out]
    n87 = call <userlib>:"TDMS Channel Write.vi"("Data"=w272, "TDMS Channel Info in"=w267) -> ()  [unwired: 9 in, 1 out]
    n88 = call <userlib>:"TDMS Channel Write.vi"("Data"=w270, "TDMS Channel Info in"=w269) -> ()  [unwired: 9 in, 1 out]
    n89 = call <userlib>:"TDMS Channel Write.vi"("Data"=w279, "TDMS Channel Info in"=w281) -> ()  [unwired: 9 in, 1 out]
    n90 = call <userlib>:"TDMS Channel Write.vi"("Data"=w280, "TDMS Channel Info in"=w282) -> ()  [unwired: 9 in, 1 out]
    n91 = node-c288() -> ()  [unwired: 1 in, 1 out]
  }
  n92 = Bundle By Name(cluster=T17 {"Yaw, Driving Straight"={"proportional gain (Kc)"=0.0, "integral time (Ti, min)"=0.0, "derivative time (Td, min)"=0.0}, "Yaw, Holding Still"={"proportional gain (Kc)"=0.0, "integral time (Ti, min)"=0.0, "derivative time (Td, min)"=0.0}, "Distance, Driving Straight"={"proportional gain (Kc)"=0.0, "integral time (Ti, min)"=0.0, "derivative time (Td, min)"=0.0}, "Distance, Holding Still"={"proportional gain (Kc)"=0.0, "integral time (Ti, min)"=0.0, "derivative time (Td, min)"=0.0}} ("PID Gains"), "Yaw, Driving Straight"=w96, "Yaw, Holding Still"=w97, "Distance, Driving Straight"=w95, "Distance, Holding Still"=w94) -> (w99:T17)
  n93 = call <userlib>:"Pneumatic Command Initialize.vi"("name (unnamed)"=w85) -> ()  [unwired: 9 in, 2 out]
  n94 = call <userlib>:"Pneumatic Command Initialize.vi"("name (unnamed)"=w77) -> ("RTFIFO Out"=w76:u64)  [unwired: 9 in, 1 out]
  n95 = call <vilib>:"WPI_SolenoidRefNum Registry Get.vi"("refnum name"="Intake Solenoid") -> ("SolenoidDevRef"=w115:T44)  [unwired: 9 in, 1 out]
  n96 = call <userlib>:"Pneumatic Command Initialize.vi"("name (unnamed)"=w85) -> ("RTFIFO Out"=w84:u64)  [unwired: 9 in, 1 out]
  n97 = call <vilib>:"WPI_SolenoidRefNum Registry Get.vi"("refnum name"="Tusks") -> ("SolenoidDevRef"=w113:T44)  [unwired: 9 in, 1 out]
  n98 = call <userlib>:"TDMS Channel Initialize.vi"("Channel"="Aliance", "Group"=w14, "TDMS"=w15) -> ("TDMS Channel Info"=w12:T11)  [unwired: 8 in]
  n99 = call <userlib>:"TDMS Channel Initialize.vi"("Channel"="Position", "Group"=w14, "TDMS"=w15) -> ("TDMS Channel Info"=w11:T11)  [unwired: 8 in]
  n100 = shared-variable ".\\Shared.lvlib\\Intake RT FIFO"(w76) -> ()  [unwired: 1 in, 1 out]
  n101 = shared-variable ".\\Shared.lvlib\\Tusks RT FIFO"(w84) -> ()  [unwired: 1 in, 1 out]
  n102 = call <userlib>:"Pneumatic Control Initialize.vi"("Forward?"=FALSE, "SolenoidDevRef"=w115, "name (unnamed)"=w77) -> ("Sense Loop"=w82:T46, "Control Loop"=w83:T48)  [unwired: 7 in]
  n103 = while {
    tunnel: w12 -> [w289]
    tunnel: w11 -> [w287]
    stop <- FALSE stop-if-true
    n104 = call <vilib>:"WPI_DriverStationGet Alliance Info.vi"() -> ("Position"=w286:T2, "Alliance"=w288:T3)  [unwired: 10 in]
    "Alliance" <- w288
    "Position" <- w286
    n105 = Wait (ms)(milliseconds to wait=u32 100) -> ()  [unwired: 1 out]
    n106 = call <userlib>:"TDMS Channel Write.vi"("Data"=w288, "TDMS Channel Info in"=w289) -> ()  [unwired: 9 in, 1 out]
    n107 = call <userlib>:"TDMS Channel Write.vi"("Data"=w286, "TDMS Channel Info in"=w287) -> ()  [unwired: 9 in, 1 out]
  }
  n108 = call <userlib>:"Drive Loop Initialize.vi"("name (unnamed)"="Drive Loop") -> ("Drive Loop Cluster"=w104:T19)  [unwired: 9 in, 1 out]
  n109 = call <vilib>:"WPI_RobotDriveRefNum Registry Get.vi"("refnum name"="driveMotors") -> ("RobotDriveDevRef"=w103:T27)  [unwired: 9 in, 1 out]
  n110 = call <userlib>:"Pneumatic Control Initialize.vi"("Forward?"=FALSE, "SolenoidDevRef"=w113, "name (unnamed)"=w85) -> ("Control Loop"=w87:T48)  [unwired: 7 in, 1 out]
  n111 = call <userlib>:"Pneumatic Control Loop.vi"("Cluster in"=w83) -> ()  [unwired: 11 in]
  n112 = call <userlib>:"Pneumatic Control Loop.vi"("Cluster in"=w87) -> ()  [unwired: 11 in]
  n113 = call <userlib>:"Pneumatic Sensor Loop.vi"("Priority"=100, "Period"=i64 20, "Solenoid Configuration"=T14 {"Normal Timing"={"Forward"=2000.0, "Reverse"=2000.0}, "Feedback Forward"=enum."Timed", "Feedback Reverse"=enum."Timed", "Analog Thresholds"={"Forward"=0.0, "Reverse"=0.0}, "Timeout"={"Forward"=0.0, "Reverse"=0.0}}, "Cluster"=w82) -> ()  [unwired: 8 in]
  n114 = call <userlib>:"Drive Loop Control Loop.vi"("Priority"=100, "Period"=i64 20, "PID Gains"=w99, "RobotDriveDevRef"=w103, "Control Cluster"=w104) -> ()  [unwired: 7 in]
  n115 = node-c288(w27) -> ()  [unwired: 1 out]
  n116 = while {
    tunnel: "AutoQCP.csv" ("File Path") -> [w297]
    i -> [w296]
    stop <- FALSE stop-if-true
    n117 = Wait (ms)(milliseconds to wait=u32 100) -> ()  [unwired: 1 out]
    n118 = Less Or Equal?(x=w296, y=10) -> (x <= y?=w294:bool)
    n119 = Or(x=w294, y="Reload QCP") -> (x .or. y?=w292:bool)
    n120 = case shown="True" w292 {
      tunnel: w297 -> [_ w301]
      frame False {
      }
      frame True {
        n121 = call "QCP Reader.vi"("Path Relative?"=TRUE, "File Path"=w301) -> ()  [unwired: 10 in]
      }
    }
  }
  n122 = call <vilib>:"WPI_EncoderRefNum Registry Get.vi"("refnum name"="Right Encoder") -> ("error out"=w120:errorcluster, "EncoderDevRef"=w121:T50)  [unwired: 9 in]
  n123 = call <userlib>:"TDMS Channel Initialize.vi"("Channel"="Right Encoder", "Group"="Auto", "TDMS"="Stronghold" ("TDMS Name")) -> ("TDMS Channel Info"=w57:T11)  [unwired: 8 in]
  n124 = call <userlib>:"Drive Loop Initialize.vi"("name (unnamed)"="Drive Loop") -> ("Numeric"=w88:u32, "Drive Loop Cluster"=w89:T19)  [unwired: 9 in]
  n125 = call <userlib>:"TDMS Channel Initialize.vi"("Channel"="Left Encoder", "Group"="Auto", "TDMS"="Stronghold" ("TDMS Name")) -> ("TDMS Channel Info"=w58:T11)  [unwired: 8 in]
  n126 = call <vilib>:"WPI_EncoderRefNum Registry Get.vi"("refnum name"="Left Encoder") -> ("error out"=w119:errorcluster, "EncoderDevRef"=w118:T50)  [unwired: 9 in]
  n127 = shared-variable ".\\Shared.lvlib\\Drive Loop RT FIFO"(w88) -> ()  [unwired: 1 in, 1 out]
  n128 = node-c288(i64 20 ("Period")) -> (w125:T23)  [unwired: 3 in]
  n129 = timed-loop "Encoder Loop" {
    timing: w125 -> [_]
    timing-out: [_] -> w124
    tunnel: w121 -> [w314]
    tunnel: w120 -> [w313]
    tunnel: w119 -> [w312]
    tunnel: w118 -> [w311]
    tunnel: w89 -> [w306]
    tunnel: w58 -> [w305]
    tunnel: w57 -> [w304]
    stop <- FALSE stop-if-true
    n130 = node-c288() -> ()  [unwired: 1 in, 1 out]
    n131 = call <vilib>:"WPI_EncoderGet.vi"("error in (no error)"=w313, "EncoderDevRef"=w314) -> ("Distance"=w302:dbl, "EncoderDevRef"=w308:T50)  [unwired: 4 in, 4 out]
    "Right Encoder Distance" <- w302
    n132 = call <vilib>:"WPI_EncoderGet.vi"("error in (no error)"=w312, "EncoderDevRef"=w311) -> ("Distance"=w303:dbl, "EncoderDevRef"=w310:T50)  [unwired: 4 in, 4 out]
    "Left Encoder Distance" <- w303
    n133 = call "Elapsed Times.vi"("Call Name"="Encoder") -> ()  [unwired: 2 in, 1 out]
    n134 = call <userlib>:"Drive Loop Encoder Count.vi"("Distance"=w303, "Drive Loop Cluster"=w306) -> ()  [unwired: 10 in]
    n135 = call <userlib>:"TDMS Channel Write.vi"("Data"=w303, "TDMS Channel Info in"=w305) -> ()  [unwired: 9 in, 1 out]
    n136 = shared-variable ".\\Shared.lvlib\\Left Encoder Distance"(w303) -> ()  [unwired: 1 in, 1 out]
    n137 = shared-variable ".\\Shared.lvlib\\Encoder Distance"(w303) -> ()  [unwired: 1 in, 1 out]
    n138 = call <userlib>:"TDMS Channel Write.vi"("Data"=w302, "TDMS Channel Info in"=w304) -> ()  [unwired: 9 in, 1 out]
    n139 = shared-variable ".\\Shared.lvlib\\Right Encoder Distance"(w302) -> ()  [unwired: 1 in, 1 out]
    n140 = case shown="True" "Reset Encoders" {
      tunnel: w310 -> [_ w317]
      tunnel: w308 -> [_ w316]
      frame False {
      }
      frame True {
        n141 = call <vilib>:"WPI_EncoderReset.vi"("EncoderDevRef"=w317) -> ()  [unwired: 9 in, 2 out]
        n142 = call <vilib>:"WPI_EncoderReset.vi"("EncoderDevRef"=w316) -> ()  [unwired: 9 in, 2 out]
      }
    }
    n143 = node-c288() -> ()  [unwired: 1 in, 1 out]
  }
  n144 = call <userlib>:"TDMS Logging Loop.vi"("Logging Period (ms)"=i64 20, "Buffer Size"=u32 1000, "Group Initialization"=T10 [{"Group"="Auto", "Channel Names"=["Auto Starting Position", "Auto Goal Target", "Auto Defense", "Robot Mode", "Auto State No Wait", "Drive CMD", "Desired Angle", "IMU Yaw", "Analog YAW Gyro", "Desired Encoder", "Left Encoder", "Right Encoder", "IMU Pitch", "Analog PITCH Gyro", "IMU Roll", "Alliance", "Position", "IMU Fault", "IMU Type", "Vision Status ", "Camera Left Target", "Camera Right Target", "Camera Target Valid", "IMU CAL M", "IMU CAL A", "IMU CAL G", "IMU CAL S", "Accel X", "Accel Y", "Accel Z"]}, {"Group"="Teleop", "Channel Names"=["Intake Roller", "Intake Solenoid"]}, {"Group"="Electrical", "Channel Names"=["PDP Voltage", "RIO Voltage"]}], "TDMS Name"="Stronghold", "Log to USB?"=FALSE) -> ()  [unwired: 7 in]
  n145 = while {
    stop <- FALSE stop-if-true
    n146 = local read "IMUStatus"() -> (w325:bool)
    n147 = shared-variable ".\\Shared.lvlib\\Sonar"() -> (w327:dbl)  [unwired: 1 in, 1 out]
    n148 = local read "Analog Pitch Gyro 2"() -> (w320:dbl)
    n149 = local read "Analog Yaw Gyro"() -> (w322:dbl)
    n150 = Wait (ms)(milliseconds to wait=u32 100) -> ()  [unwired: 1 out]
    n151 = shared-variable ".\\Shared.lvlib\\Right Encoder Distance"() -> (w330:dbl)  [unwired: 1 in, 1 out]
    n152 = shared-variable ".\\Shared.lvlib\\Left Encoder Distance"() -> (w332:dbl)  [unwired: 1 in, 1 out]
    n153 = shared-variable ".\\Shared.lvlib\\IMU Yaw"() -> (w329:dbl)  [unwired: 1 in, 1 out]
    n154 = call-poly <vilib>:"NT Write Value.vi"("Numeric"=w327, "Name"="Sharp Sensor") -> ()  [unwired: 9 in, 1 out]
    n155 = call-poly <vilib>:"NT Write Value.vi"("Boolean"=w325, "Name"="IMU Error") -> ()  [unwired: 9 in, 1 out]
    n156 = call-poly <vilib>:"NT Write Value.vi"("Numeric"=w320, "Name"="Analog Pitch Gyro") -> ()  [unwired: 9 in, 1 out]
    n157 = call-poly <vilib>:"NT Write Value.vi"("Numeric"=w322, "Name"="Analog Yaw Gyro") -> ()  [unwired: 9 in, 1 out]
    n158 = call-poly <vilib>:"NT Write Value.vi"("Numeric"=w332, "Name"="Left Encoder") -> ()  [unwired: 9 in, 1 out]
    n159 = call-poly <vilib>:"NT Write Value.vi"("Numeric"=w330, "Name"="Right Encoder") -> ()  [unwired: 9 in, 1 out]
    n160 = call-poly <vilib>:"NT Write Value.vi"("Numeric"=w329, "Name"="IMU Yaw") -> ()  [unwired: 9 in, 1 out]
  }
  n161 = node-c288(w124) -> ()  [unwired: 1 out]
  n162 = call <userlib>:"TDMS Channel Initialize.vi"("Channel"="Analog Gyro Yaw", "Group"=w32, "TDMS"=w33) -> ("TDMS Channel Info"=w35:T11)  [unwired: 8 in]
  n163 = call <userlib>:"TDMS Channel Initialize.vi"("Channel"="Analog Gyro Pitch", "Group"=w32, "TDMS"=w33) -> ("TDMS Channel Info"=w38:T11)  [unwired: 8 in]
  n164 = call <userlib>:"TDMS Channel Initialize.vi"("Channel"="IMU Yaw", "Group"=w32, "TDMS"=w33) -> ("TDMS Channel Info"=w66:T11)  [unwired: 8 in]
  n165 = call <userlib>:"TDMS Channel Initialize.vi"("Channel"="IMU Pitch", "Group"=w32, "TDMS"=w33) -> ("TDMS Channel Info"=w65:T11)  [unwired: 8 in]
  n166 = call <userlib>:"TDMS Channel Initialize.vi"("Channel"="IMU Roll", "Group"=w32, "TDMS"=w33) -> ("TDMS Channel Info"=w64:T11)  [unwired: 8 in]
  n167 = call <userlib>:"TDMS Channel Initialize.vi"("Channel"="Accel X", "Group"=w32, "TDMS"=w33) -> ("TDMS Channel Info"=w51:T11)  [unwired: 8 in]
  n168 = call <userlib>:"TDMS Channel Initialize.vi"("Channel"="Accel Y", "Group"=w32, "TDMS"=w33) -> ("TDMS Channel Info"=w50:T11)  [unwired: 8 in]
  n169 = call <userlib>:"TDMS Channel Initialize.vi"("Channel"="Accel Z", "Group"=w32, "TDMS"=w33) -> ("TDMS Channel Info"=w49:T11)  [unwired: 8 in]
  n170 = call <userlib>:"TDMS Channel Initialize.vi"("Channel"="IMU Cal M", "Group"=w32, "TDMS"=w33) -> ("TDMS Channel Info"=w44:T11)  [unwired: 8 in]
  n171 = call <userlib>:"TDMS Channel Initialize.vi"("Channel"="IMU Cal A", "Group"=w32, "TDMS"=w33) -> ("TDMS Channel Info"=w43:T11)  [unwired: 8 in]
  n172 = call <userlib>:"TDMS Channel Initialize.vi"("Channel"="IMU Cal G", "Group"=w32, "TDMS"=w33) -> ("TDMS Channel Info"=w42:T11)  [unwired: 8 in]
  n173 = call <userlib>:"TDMS Channel Initialize.vi"("Channel"="IMU Cal S", "Group"=w32, "TDMS"=w33) -> ("TDMS Channel Info"=w41:T11)  [unwired: 8 in]
  n174 = call <userlib>:"TDMS Channel Initialize.vi"("Channel"="IMU Type", "Group"=w32, "TDMS"=w33) -> ("TDMS Channel Info"=w31:T11)  [unwired: 8 in]
  n175 = call <userlib>:"TDMS Channel Initialize.vi"("Channel"="IMU Stats", "Group"=w32, "TDMS"=w33) -> ("TDMS Channel Info"=w39:T11)  [unwired: 8 in]
  n176 = Bundle By Name(cluster=T13 {"IMU Yaw"={"TDMS Data"={"Group/CMD"=0, "Channel"=0, "Data"=0.0}, "TDMS RT FIFO"=refnum}, "IMU Pitch"={"TDMS Data"={"Group/CMD"=0, "Channel"=0, "Data"=0.0}, "TDMS RT FIFO"=refnum}, "IMU Roll"={"TDMS Data"={"Group/CMD"=0, "Channel"=0, "Data"=0.0}, "TDMS RT FIFO"=refnum}, "Accel X"={"TDMS Data"={"Group/CMD"=0, "Channel"=0, "Data"=0.0}, "TDMS RT FIFO"=refnum}, "Accel Y"={"TDMS Data"={"Group/CMD"=0, "Channel"=0, "Data"=0.0}, "TDMS RT FIFO"=refnum}, "Accel Z"={"TDMS Data"={"Group/CMD"=0, "Channel"=0, "Data"=0.0}, "TDMS RT FIFO"=refnum}, "IMU Cal M"={"TDMS Data"={"Group/CMD"=0, "Channel"=0, "Data"=0.0}, "TDMS RT FIFO"=refnum}, "IMU Cal A"={"TDMS Data"={"Group/CMD"=0, "Channel"=0, "Data"=0.0}, "TDMS RT FIFO"=refnum}, "IMU Cal G"={"TDMS Data"={"Group/CMD"=0, "Channel"=0, "Data"=0.0}, "TDMS RT FIFO"=refnum}, "IMU Cal S"={"TDMS Data"={"Group/CMD"=0, "Channel"=0, "Data"=0.0}, "TDMS RT FIFO"=refnum}, "IMU Type"={"TDMS Data"={"Group/CMD"=0, "Channel"=0, "Data"=0.0}, "TDMS RT FIFO"=refnum}}, "IMU Yaw"=w66, "IMU Pitch"=w65, "IMU Roll"=w64, "Accel X"=w51, "Accel Y"=w50, "Accel Z"=w49, "IMU Cal M"=w44, "IMU Cal A"=w43, "IMU Cal G"=w42, "IMU Cal S"=w41, "IMU Type"=w31) -> (w63:T13)
  n177 = call <userlib>:"Drive Loop Initialize.vi"("name (unnamed)"="Drive Loop") -> ("Drive Loop Cluster"=w91:T19)  [unwired: 9 in, 1 out]
  n178 = call <vilib>:"WPI_GyroRefNum Registry Get.vi"("refnum name"="Pitch Gyro") -> ("GyroDevRef"=w111:T54)  [unwired: 9 in, 1 out]
  n179 = call "IMUOrientRefNum Registry Get.vi"("refnum name"="Alt IMU") -> ("I2CDevRef out"=w106:T57)  [unwired: 9 in, 1 out]
  n180 = call "IMUOrientRefNum Registry Get.vi"("refnum name"="Pri IMU") -> ("I2CDevRef out"=w116:T57)  [unwired: 9 in, 1 out]
  n181 = call <vilib>:"WPI_GyroRefNum Registry Get.vi"("refnum name"="Gyro") -> ("GyroDevRef"=w127:T54)  [unwired: 9 in, 1 out]
  n182 = node-c288() -> (w131:T23)  [unwired: 4 in]
  n183 = timed-loop "IMU Loop, Time Critical" {
    timing: w131 -> [_]
    timing-out: [_] -> w130
    tunnel: w116 -> [w373]
    tunnel: w127 -> [w371]
    tunnel: w111 -> [w369]
    shift-right: [w336] -> _
    shift-left: IMUType."Pri IMU" -> [w367]
    shift-right: [w366] -> _
    shift-left: T18 {"Yaw Wind"=0.0, "Roll Wind"=0.0, "Pitch Wind"=0.0} -> [w365]
    tunnel: w106 -> [w364]
    tunnel: w91 -> [w361]
    tunnel: w63 -> [w354]
    tunnel: w39 -> [w345]
    tunnel: w38 -> [w340]
    tunnel: w35 -> [w338]
    stop <- _ stop-if-true
    n184 = node-c288() -> (→"Late? 2":bool)  [unwired: 1 in]
    n185 = Unbundle By Name(w373) -> ("DevStatus.status"=w342:bool)
    "IMUStatus" <- w342
    n186 = call "Elapsed Times.vi"("Call Name"="IMU") -> ()  [unwired: 2 in, 1 out]
    n187 = call <vilib>:"WPI_GyroGetAngle.vi"("GyroDevRef"=w369) -> ("Angle"=w368:dbl)  [unwired: 6 in, 4 out]
    n188 = call <vilib>:"WPI_GyroGetAngle.vi"("GyroDevRef"=w371) -> ("Angle"=w370:dbl)  [unwired: 6 in, 4 out]
    n189 = Negate(x=w368) -> (-x=w341:dbl)
    "Analog Pitch Gyro 2" <- w341
    n190 = Boolean To (0,1)(Boolean=w342) -> (0, 1=w344:i16)
    n191 = call <userlib>:"TDMS Channel Write.vi"("Data"=w341, "TDMS Channel Info in"=w340) -> ()  [unwired: 9 in, 1 out]
    n192 = case shown="\"Pri IMU\", Default" w367 {
      selector: w367 -> [w403 w457 _]
      tunnel: w373 -> [w424 _ _]
      tunnel: [w413 w467 w484] -> w359
      tunnel: w370 -> [w390 w443 w489]
      tunnel: [w388 w441 w483] -> w357
      tunnel: w341 -> [_ _ w488]
      tunnel: [w404 w458 IMUType."Analog GYRO"] -> w336
      tunnel: [w396 w450 _] -> w366
      tunnel: w365 -> [w395 w449 w487]
      tunnel: w364 -> [_ w444 _]
      tunnel: [w390 w443 w484] -> w339
      tunnel: [w389 w442 w484] -> w363
      tunnel: [w388 w441 w483] -> w362
      tunnel: [w387 w440 0.0 ("Pitch Wind")] -> w355
      tunnel: w354 -> [w386 w439 _]
      tunnel: [w376 w432 _] -> w349
      tunnel: [w377 w431 _] -> w348
      tunnel: [w378 w430 _] -> w347
      tunnel: [w379 w429 _] -> w346
      frame "Pri IMU", Default {
        n193 = First Call?() -> (First Call?: T/F=w394:bool)
        n194 = call "IMUOrientRead.vi"("I2CDevRef"=w424, "Orient Reset"=w394, "Read Enable"="Read Enable", "Orient Ref"=w395, "Earth Field (uT)"="Earth Field (uT)") -> ("Cal Status"=w427:T59, "Orient Y/R/P"=w397:T60, "Acc X,Y,Z"=w426:cluster{"X Acc":dbl, "Y Acc":dbl, "Z Acc":dbl}, "Mag Field X,Y,Z"=w414:T61)  [unwired: 4 in, 3 out]
        n195 = Unbundle By Name(w397) -> ("Yaw Wind"=w400:dbl, "Roll Wind"=w399:dbl, "Pitch Wind"=w398:dbl)
        n196 = Unbundle By Name(w414) -> ("X Mag"=w416:dbl, "Y Mag"=w417:dbl, "Z Mag"=w418:dbl, "Anomaly"=→"Anomaly":bool)
        n197 = Unbundle By Name(w386) -> ("Accel X"=w385:T11, "Accel Y"=w384:T11, "Accel Z"=w383:T11)
        n198 = Unbundle By Name(w426) -> ("X Acc"=w382:dbl, "Y Acc"=w381:dbl, "Z Acc"=w380:dbl)
        "X Acc" <- w382
        "Y Acc" <- w381
        "Z Acc" <- w380
        n199 = Unbundle(w427) -> ("Mag"=w412:T62, "Acc"=w407:T62, "Gyro"=w406:T62, "Sys"=w405:T62, "Status"=w402:bool)
        "S" <- w405
        "G" <- w406
        "A" <- w407
        "M" <- w412
        n200 = call <userlib>:"TDMS Channel Write.vi"("Data"=w382, "TDMS Channel Info in"=w385) -> ()  [unwired: 9 in, 1 out]
        n201 = call <userlib>:"TDMS Channel Write.vi"("Data"=w381, "TDMS Channel Info in"=w384) -> ()  [unwired: 9 in, 1 out]
        n202 = call <userlib>:"TDMS Channel Write.vi"("Data"=w380, "TDMS Channel Info in"=w383) -> ()  [unwired: 9 in, 1 out]
        n203 = shared-variable ".\\Shared.lvlib\\Accel X"(w382) -> ()  [unwired: 1 in, 1 out]
        n204 = shared-variable ".\\Shared.lvlib\\Accel Y"(w381) -> ()  [unwired: 1 in, 1 out]
        n205 = shared-variable ".\\Shared.lvlib\\Accel Z"(w380) -> ()  [unwired: 1 in, 1 out]
        n206 = Cluster To Array(cluster=w412) -> (array=w411:bool[])
        n207 = Cluster To Array(cluster=w407) -> (array=w410:bool[])
        n208 = Cluster To Array(cluster=w406) -> (array=w409:bool[])
        n209 = Cluster To Array(cluster=w405) -> (array=w408:bool[])
        n210 = Square(x=w416) -> (x^2=w420:dbl)
        n211 = Square(x=w417) -> (x^2=w421:dbl)
        n212 = Square(x=w418) -> (x^2=w419:dbl)
        n213 = Not(x=w402) -> (.not. x?=w391:bool)
        n214 = Unbundle By Name(w397) -> ("Yaw Wind"=w413:dbl, "Yaw Wind"=w389:dbl, "Roll Wind"=w388:dbl, "Pitch Wind"=w387:dbl)
        "pitch" <- w388
        n215 = Compound Arithmetic op=ADD(w419, w420, w421) -> (w422:dbl)
        n216 = Boolean Array To Number(Boolean array=w411) -> (number=w379:u32)
        n217 = Boolean Array To Number(Boolean array=w410) -> (number=w378:u32)
        n218 = Boolean Array To Number(Boolean array=w409) -> (number=w377:u32)
        n219 = Boolean Array To Number(Boolean array=w408) -> (number=w376:u32)
        n220 = shared-variable ".\\Shared.lvlib\\IMU Cal M"(w379) -> ()  [unwired: 1 in, 1 out]
        n221 = shared-variable ".\\Shared.lvlib\\IMU Cal A"(w378) -> ()  [unwired: 1 in, 1 out]
        n222 = shared-variable ".\\Shared.lvlib\\IMU Cal G"(w377) -> ()  [unwired: 1 in, 1 out]
        n223 = shared-variable ".\\Shared.lvlib\\IMU Cal S"(w376) -> ()  [unwired: 1 in, 1 out]
        n224 = Or(x="PImu fail", y=w391) -> (x .or. y?=w393:bool)
        n225 = Square Root(x=w422) -> (sqrt(x)=→"Mag Vector":dbl)
        n226 = Select(t=IMUType."Alt IMU", s=w393, f=w403) -> (s? t:f=w404:T1)
        n227 = shared-variable ".\\Shared.lvlib\\IMU Roll"(w387) -> ()  [unwired: 1 in, 1 out]
        n228 = Bundle("Yaw Wind"=w400, "Roll Wind"=w399, "Pitch Wind"=w398) -> (w396:T18)  [unwired: 1 in]
      }
      frame "Alt IMU" {
        n229 = First Call?() -> (First Call?: T/F=w448:bool)
        n230 = call "IMUOrientRead.vi"("I2CDevRef"=w444, "Orient Reset"=w448, "Read Enable"="Read Enable 2", "Orient Ref"=w449, "Earth Field (uT)"="Earth Field (uT) 2") -> ("Cal Status"=w480:T59, "Orient Y/R/P"=w451:T60, "Acc X,Y,Z"=w479:cluster{"X Acc":dbl, "Y Acc":dbl, "Z Acc":dbl}, "Mag Field X,Y,Z"=w468:T61)  [unwired: 4 in, 3 out]
        n231 = Unbundle By Name(w451) -> ("Yaw Wind"=w454:dbl, "Roll Wind"=w453:dbl, "Pitch Wind"=w452:dbl)
        n232 = Unbundle By Name(w468) -> ("X Mag"=w470:dbl, "Y Mag"=w471:dbl, "Z Mag"=w472:dbl, "Anomaly"=→"Anomaly 2":bool)
        n233 = Unbundle By Name(w439) -> ("Accel X"=w438:T11, "Accel Y"=w437:T11, "Accel Z"=w436:T11)
        n234 = Unbundle By Name(w479) -> ("X Acc"=w435:dbl, "Y Acc"=w434:dbl, "Z Acc"=w433:dbl)
        "X Acc 2" <- w435
        "Y Acc 2" <- w434
        "Z Acc 2" <- w433
        n235 = Unbundle(w480) -> ("Mag"=w466:T62, "Acc"=w461:T62, "Gyro"=w460:T62, "Sys"=w459:T62, "Status"=w456:bool)
        "S 2" <- w459
        "G 2" <- w460
        "A 2" <- w461
        "M 2" <- w466
        n236 = call <userlib>:"TDMS Channel Write.vi"("Data"=w435, "TDMS Channel Info in"=w438) -> ()  [unwired: 9 in, 1 out]
        n237 = call <userlib>:"TDMS Channel Write.vi"("Data"=w434, "TDMS Channel Info in"=w437) -> ()  [unwired: 9 in, 1 out]
        n238 = call <userlib>:"TDMS Channel Write.vi"("Data"=w433, "TDMS Channel Info in"=w436) -> ()  [unwired: 9 in, 1 out]
        n239 = Square(x=w470) -> (x^2=w474:dbl)
        n240 = Square(x=w471) -> (x^2=w475:dbl)
        n241 = Square(x=w472) -> (x^2=w473:dbl)
        n242 = Unbundle By Name(w451) -> ("Yaw Wind"=w467:dbl, "Yaw Wind"=w442:dbl, "Roll Wind"=w441:dbl, "Pitch Wind"=w440:dbl)
        "pitch 2" <- w441
        n243 = shared-variable ".\\Shared.lvlib\\Accel X"(w435) -> ()  [unwired: 1 in, 1 out]
        n244 = shared-variable ".\\Shared.lvlib\\Accel Y"(w434) -> ()  [unwired: 1 in, 1 out]
        n245 = shared-variable ".\\Shared.lvlib\\Accel Z"(w433) -> ()  [unwired: 1 in, 1 out]
        n246 = Compound Arithmetic op=ADD(w473, w474, w475) -> (w476:dbl)
        n247 = Cluster To Array(cluster=w466) -> (array=w465:bool[])
        n248 = Cluster To Array(cluster=w461) -> (array=w464:bool[])
        n249 = Cluster To Array(cluster=w460) -> (array=w463:bool[])
        n250 = Cluster To Array(cluster=w459) -> (array=w462:bool[])
        n251 = Not(x=w456) -> (.not. x?=w445:bool)
        n252 = Boolean Array To Number(Boolean array=w465) -> (number=w429:u32)
        n253 = Boolean Array To Number(Boolean array=w464) -> (number=w430:u32)
        n254 = Boolean Array To Number(Boolean array=w463) -> (number=w431:u32)
        n255 = Boolean Array To Number(Boolean array=w462) -> (number=w432:u32)
        n256 = Square Root(x=w476) -> (sqrt(x)=→"Mag Vector 2":dbl)
        n257 = Or(x=w445, y="Alt imu") -> (x .or. y?=w447:bool)
        n258 = shared-variable ".\\Shared.lvlib\\IMU Cal M"(w429) -> ()  [unwired: 1 in, 1 out]
        n259 = shared-variable ".\\Shared.lvlib\\IMU Cal A"(w430) -> ()  [unwired: 1 in, 1 out]
        n260 = shared-variable ".\\Shared.lvlib\\IMU Cal G"(w431) -> ()  [unwired: 1 in, 1 out]
        n261 = shared-variable ".\\Shared.lvlib\\IMU Cal S"(w432) -> ()  [unwired: 1 in, 1 out]
        n262 = shared-variable ".\\Shared.lvlib\\IMU Roll"(w440) -> ()  [unwired: 1 in, 1 out]
        n263 = Select(t=IMUType."Analog GYRO", s=w447, f=w457) -> (s? t:f=w458:T1)
        n264 = Bundle("Yaw Wind"=w454, "Roll Wind"=w453, "Pitch Wind"=w452) -> (w450:T18)  [unwired: 1 in]
      }
      frame "Analog GYRO" {
        n265 = Unbundle By Name(w487) -> ("Yaw Wind"=w486:dbl, "Roll Wind"=w485:dbl)  [unwired: 1 out]
        n266 = Subtract(x=w488, y=w485) -> (x-y=w492:dbl)
        n267 = Subtract(x=w489, y=w486) -> (x-y=w495:dbl)
        n268 = feedback #1() -> (w491:dbl)  [unwired: 1 in]
        n269 = feedback #2() -> (w496:dbl)  [unwired: 1 in]
        n270 = First Call?() -> (First Call?: T/F=w493:bool)
        n271 = First Call?() -> (First Call?: T/F=w494:bool)
        n272 = Select(t=w492, s=w493, f=w491) -> (s? t:f=w490:dbl)
        n273 = feedback-in #1(w490) -> ()
        n274 = Select(t=w495, s=w494, f=w496) -> (s? t:f=w497:dbl)
        n275 = feedback-in #2(w497) -> ()
        n276 = Subtract(x=w488, y=w490) -> (x-y=w483:dbl)
        n277 = Subtract(x=w489, y=w497) -> (x-y=w484:dbl)
      }
    }
    "Analog Yaw Gyro" <- w339
    "Yaw" <- w363
    "Pitch" <- w362
    "Roll" <- w355
    "IMU Type" <- w336
    n278 = To Double Precision Float(number=w344) -> (double precision float=w343:dbl)
    n279 = call <userlib>:"TDMS Channel Write.vi"("Data"=w343, "TDMS Channel Info in"=w345) -> ()  [unwired: 9 in, 1 out]
    n280 = Unbundle By Name(w354) -> ("IMU Cal M"=w353:T11, "IMU Cal A"=w352:T11, "IMU Cal G"=w351:T11, "IMU Cal S"=w350:T11, "IMU Type"=w337:T11)
    n281 = Unbundle By Name(w354) -> ("IMU Yaw"=w360:T11, "IMU Pitch"=w358:T11, "IMU Roll"=w356:T11)
    n282 = call <userlib>:"TDMS Channel Write.vi"("Data"=w339, "TDMS Channel Info in"=w338) -> ()  [unwired: 9 in, 1 out]
    n283 = call <userlib>:"Drive Loop Gyro Angle.vi"("Yaw Wind"=w359, "Drive Loop Cluster"=w361) -> ()  [unwired: 10 in]
    n284 = call <userlib>:"TDMS Channel Write.vi"("Data"=w359, "TDMS Channel Info in"=w360) -> ()  [unwired: 9 in, 1 out]
    n285 = call <userlib>:"TDMS Channel Write.vi"("Data"=w357, "TDMS Channel Info in"=w358) -> ()  [unwired: 9 in, 1 out]
    n286 = call <userlib>:"TDMS Channel Write.vi"("Data"=w355, "TDMS Channel Info in"=w356) -> ()  [unwired: 9 in, 1 out]
    n287 = call <userlib>:"TDMS Channel Write.vi"("Data"=w346, "TDMS Channel Info in"=w353) -> ()  [unwired: 9 in, 1 out]
    n288 = call <userlib>:"TDMS Channel Write.vi"("Data"=w347, "TDMS Channel Info in"=w352) -> ()  [unwired: 9 in, 1 out]
    n289 = call <userlib>:"TDMS Channel Write.vi"("Data"=w348, "TDMS Channel Info in"=w351) -> ()  [unwired: 9 in, 1 out]
    n290 = call <userlib>:"TDMS Channel Write.vi"("Data"=w349, "TDMS Channel Info in"=w350) -> ()  [unwired: 9 in, 1 out]
    n291 = call <userlib>:"TDMS Channel Write.vi"("Data"=w336, "TDMS Channel Info in"=w337) -> ()  [unwired: 9 in, 1 out]
    n292 = shared-variable ".\\Shared.lvlib\\IMU Yaw"(w359) -> ()  [unwired: 1 in, 1 out]
    n293 = shared-variable ".\\Shared.lvlib\\IMU Pitch"(w357) -> ()  [unwired: 1 in, 1 out]
    n294 = node-c288("Sensor Period") -> ()  [unwired: 1 out]
  }
  n295 = node-c288(w130) -> ()  [unwired: 1 out]
